vi "Get SelectorTunnel Terminals.vi"(8 "error in (no error)":errorcluster, 11 "SelectorTunnel in":refnum<vi>) -> (0 "error out":errorcluster, 1 "Outside Terminal":refnum<vi>, 2 "Inside Terminals[]":refnum<vi>[](array[refnum]), 3 "SelectorTunnel out":refnum<vi>)   [LabVIEW 2014]
doc: "Returns inner terminal array for LoopTunnel and outer terminal."
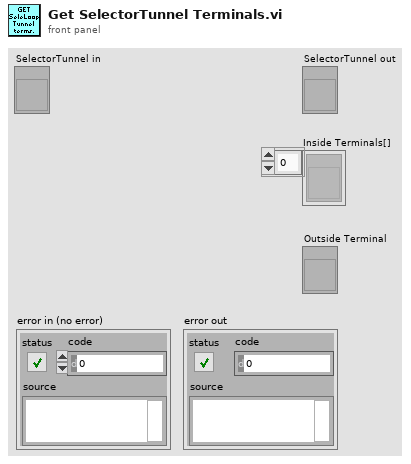
[diagram p1: front panel]
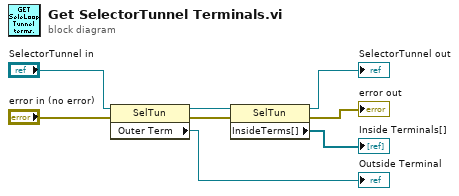
[diagram p0: block diagram]
diagram:
  n1 = property class="SelTun"(reference="SelectorTunnel in", error in="error in (no error)") -> (reference out=w2:refnum<vi>, error out=w6:errorcluster, "Outer Term"=→"Outside Terminal":refnum<vi>)
  n2 = property class="SelTun"(reference=w2, error in=w6) -> (reference out=→"SelectorTunnel out":refnum<vi>, error out=→"error out":errorcluster, "InsideTerms[]"=→"Inside Terminals[]":refnum<vi>[])
